vi "HXG2_PIDs.vi"(6 "PID Ctrls":T1, 7 "Analog In":T2, 8 "error in (no error)":errorcluster, 9 "AIR-LIQ Cluster":T4 {"Liq Cluster"."Liq TEMP %" min=0.0 max=100.0 step=1.0 format="%#.1f"; "Liq Cluster"."Liq FLOW %" min=0.0 max=100.0 step=1.0 format="%#.1f"; "Liq Cluster"."TLiq °F" min=40.0 max=180.0 step=1.0 format="%#.1f"; "Liq Cluster"."Mdot lbm/hr" min=0.0 max=1000.0 step=1.0 format="%#.1f"; "Air Cluster"."Air TEMP %" min=0.0 max=100.0 step=1.0 format="%#.1f"; "Air Cluster"."Air FLOW %" min=0.0 max=100.0 step=1.0 format="%#.1f"; "Air Cluster"."Tair  °F" min=-5.0 max=100.0 step=1.0 format="%#.1f"; "Air Cluster"."CFMs" min=0.0 max=200.0 step=1.0 format="%#.1f"}, 10 "PID Cluster":T7, 11 "Calculated Values":T3) -> (0 "error out":errorcluster, 3 "PID Ctrls Out":T1)   [LabVIEW 2012]
uses:
  <vilib>/addons/control/pid/NI_PID_pid.lvlib
  <vilib>/addons/control/pid/pid.llb/PID Control Input Filter (DBL).vi
  <vilib>/addons/control/pid/pid.llb/PID Advanced (DBL).vi
  Controls/UI/HXG2_NumDisplayLarge.ctl
  Modules/EnableAirGly/HXG2enable.ctl
  <vilib>/addons/control/pid/pid.llb/PID Gain Schedule (DBL).vi
  <vilib>/addons/control/pid/pid.llb/PID Structure Conversion (DBL).vi
  Controls/HXG2_PIDctrlsOUT.ctl
  Controls/HXG2_PIDon-off.ctl
  Controls/HXG2_PIDCluster.ctl
  Controls/UI/HXG2_UI_ControlSetAir.ctl
  Controls/UI/HXG2_UI_ControlSetGly.ctl
  Controls/HXG2_AirGly-Cluster.ctl
  Controls/HXG2_Calculated.ctl
  Controls/HXG2_AnalogIn.ctl
  Controls/HXG2_AirPIDresets.ctl
  Controls/HXG2_LiqPIDresets.ctl
  Controls/HXG2_PIDgains_SchedulingArray_BasicBlock.ctl
  Controls/HXG2_PIDgains_SchedulingArray.ctl
  Controls/HXG2_PIDgains_SchedulingArrayWITHLimits.ctl
panel:
  out "PID Air Heat":dbl format="%.2f"
  out "FFAir Heat":dbl
  in  "Lheat range":cluster{"setpoint high":dbl, "setpoint low":dbl}={"setpoint high"=100.0, "setpoint low"=0.0} {"setpoint high" format="%.2f"; "setpoint low" format="%.2f"}
  in  "Lcool range":cluster{"setpoint high":dbl, "setpoint low":dbl}={"setpoint high"=100.0, "setpoint low"=0.0} {"setpoint high" format="%.2f"; "setpoint low" format="%.2f"}
  out "Current State":i32
  in  "Lflow range":cluster{"setpoint high":dbl, "setpoint low":dbl}={"setpoint high"=100.0, "setpoint low"=0.0} {"setpoint high" format="%.2f"; "setpoint low" format="%.2f"}
  in  "Aheat range":cluster{"setpoint high":dbl, "setpoint low":dbl}={"setpoint high"=100.0, "setpoint low"=0.0} {"setpoint high" format="%.2f"; "setpoint low" format="%.2f"}
  in  "Acool range":cluster{"setpoint high":dbl, "setpoint low":dbl}={"setpoint high"=100.0, "setpoint low"=0.0} {"setpoint high" format="%.2f"; "setpoint low" format="%.2f"}
  in  "Aflow range":cluster{"setpoint high":dbl, "setpoint low":dbl}={"setpoint high"=100.0, "setpoint low"=0.0} {"setpoint high" format="%.2f"; "setpoint low" format="%.2f"}
  out "dt out (s)":dbl format="%.3f"
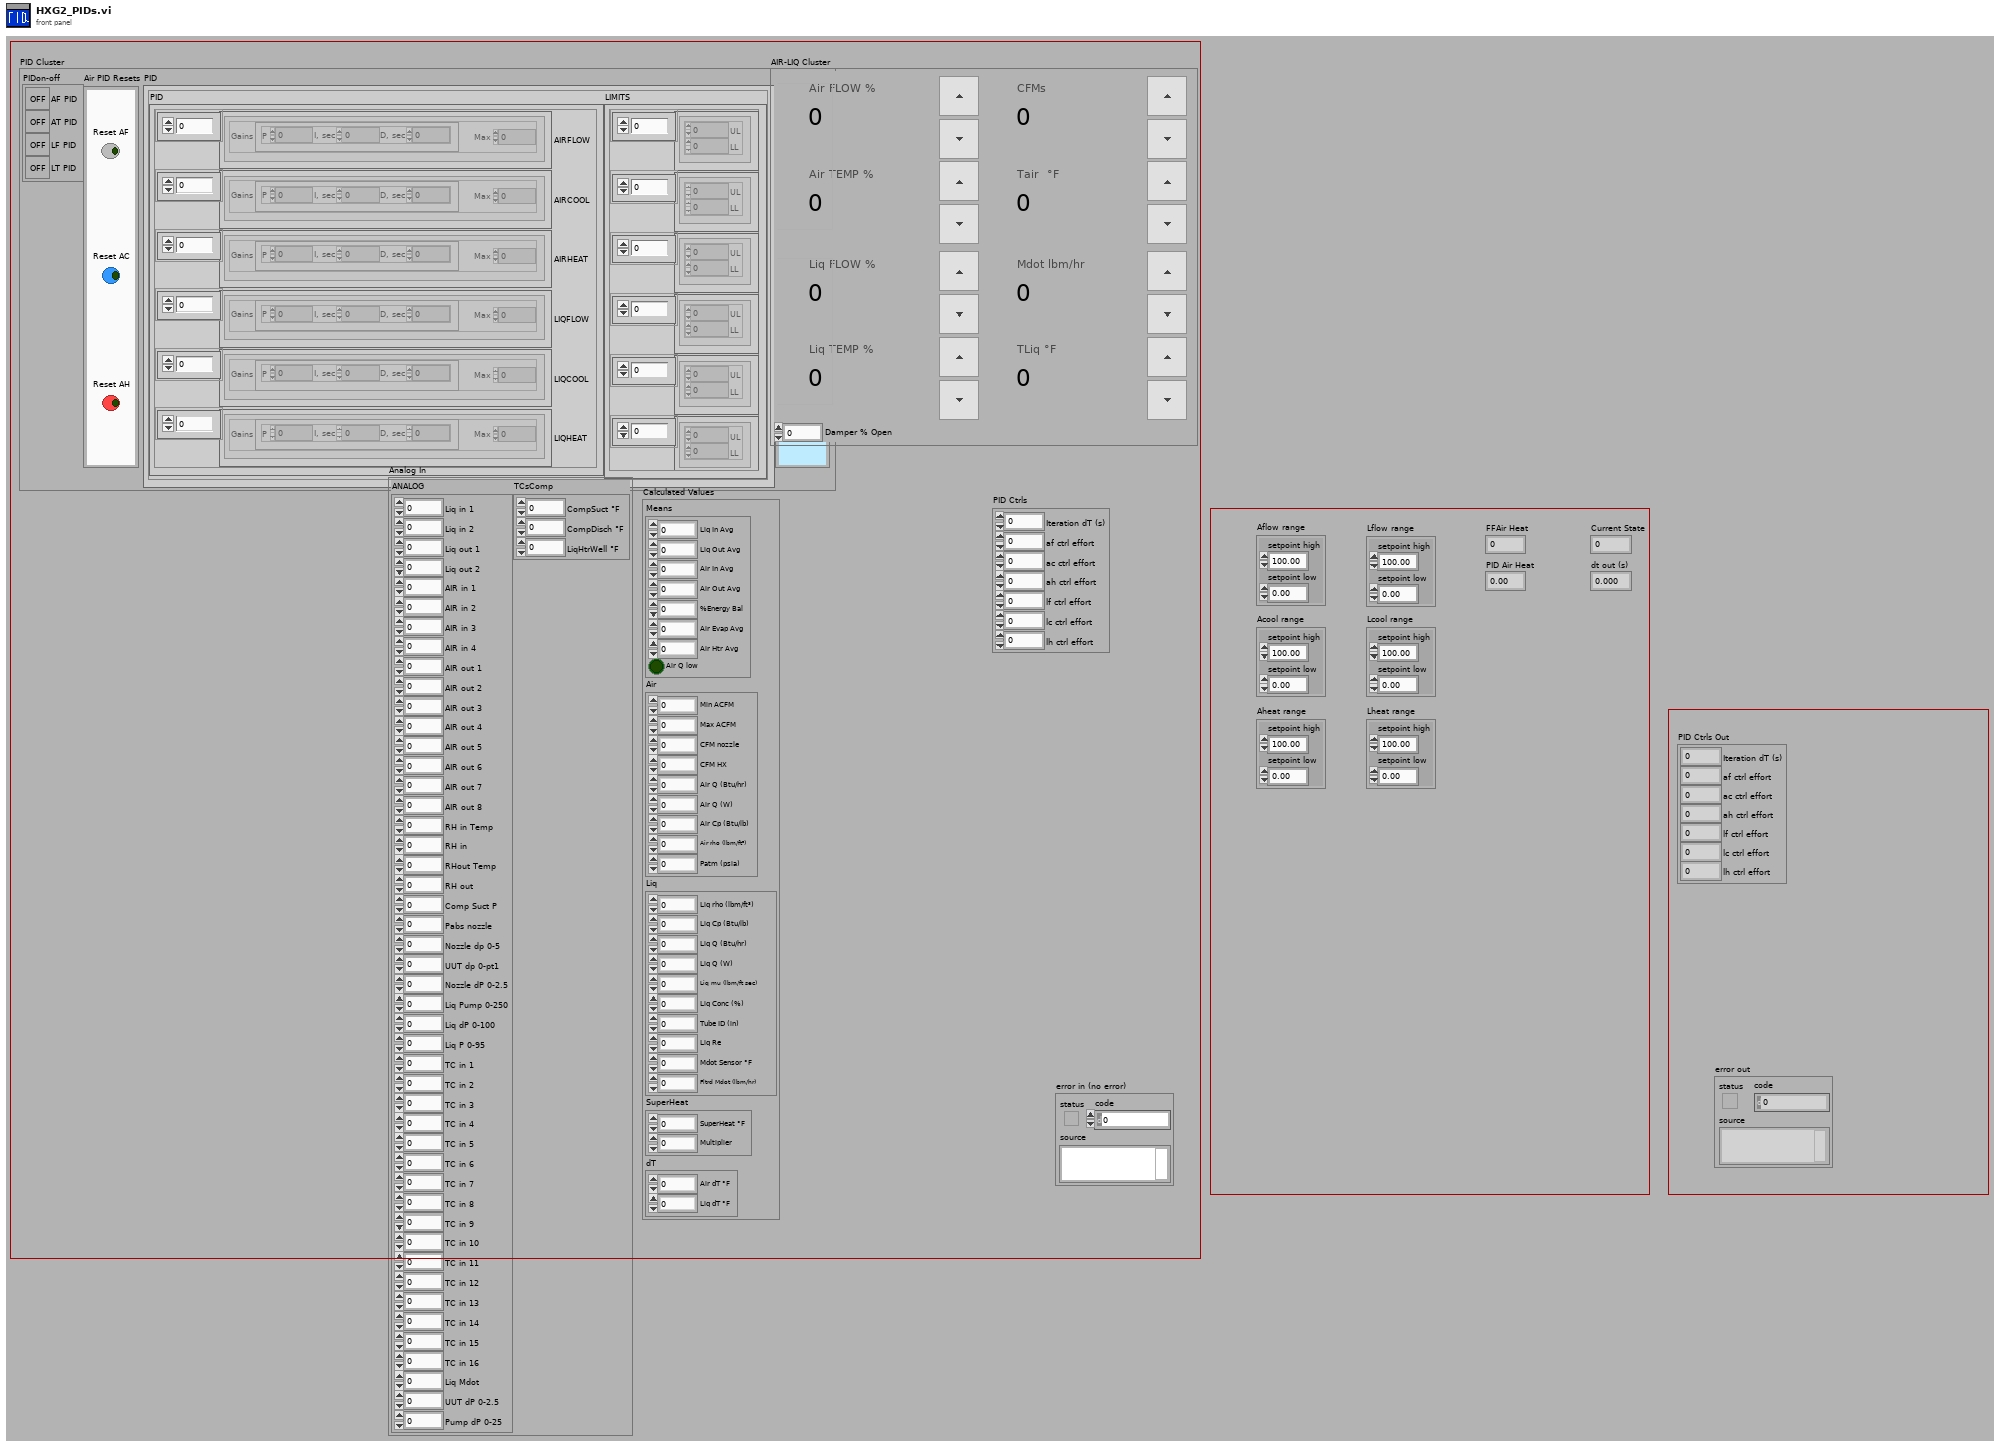
[diagram p1: front panel]
types:
  T1 = typedef "HXG2_PIDctrlsOUT.ctl" = cluster{"Iteration dT (s)":dbl, "af ctrl effort":dbl, "ac ctrl effort":dbl, "ah ctrl effort":dbl, "lf ctrl effort":dbl, "lc ctrl effort":dbl, "lh ctrl effort":dbl}
  T2 = typedef "HXG2_AnalogIn.ctl" = cluster{"ANALOG":cluster{"Liq in 1":dbl, "Liq in 2":dbl, "Liq out 1":dbl, "Liq out 2":dbl, "AIR in 1":dbl, "AIR in 2":dbl, "AIR in 3":dbl, "AIR in 4":dbl, "AIR out 1":dbl, "AIR out 2":dbl, "AIR out 3":dbl, "AIR out 4":dbl, "AIR out 5":dbl, "AIR out 6":dbl, "AIR out 7":dbl, "AIR out 8":dbl, "RH in Temp":dbl, "RH in":dbl, "RHout Temp":dbl, "RH out":dbl, "Comp Suct P":dbl, "Pabs nozzle":dbl, "Nozzle dp 0-5":dbl, "UUT dp 0-pt1":dbl, "Nozzle dP 0-2.5":dbl, "Liq Pump 0-250":dbl, "Liq dP 0-100":dbl, "Liq P 0-95":dbl, "TC in 1":dbl, "TC in 2":dbl, "TC in 3":dbl, "TC in 4":dbl, "TC in 5":dbl, "TC in 6":dbl, "TC in 7":dbl, "TC in 8":dbl, "TC in 9":dbl, "TC in 10":dbl, "TC in 11":dbl, "TC in 12":dbl, "TC in 13":dbl, "TC in 14":dbl, "TC in 15":dbl, "TC in 16":dbl, "Liq Mdot":dbl, "UUT dP 0-2.5":dbl, "Pump dP 0-25":dbl}, "TCsComp":cluster{"CompSuct °F  ":dbl, "CompDisch °F":dbl, "LiqHtrWell °F":dbl}}
  T3 = typedef "HXG2_Calculated.ctl" = cluster{"Means":cluster{"Liq In Avg":dbl, "Liq Out Avg":dbl, "Air In Avg":dbl, "Air Out Avg":dbl, "%Energy Bal":dbl, "Air Evap Avg":dbl, "Air Htr Avg":dbl, "Air Q low":bool}, "Air":cluster{"Min ACFM":dbl, "Max ACFM":dbl, "CFM nozzle":dbl, "CFM HX":dbl, "Air Q (Btu/hr)":dbl, "Air Q (W)":dbl, "Air Cp (Btu/lb)":dbl, "Air rho (lbm/ft³)":dbl, "Patm (psia)":dbl}, "Liq":cluster{"Liq rho (lbm/ft³)":dbl, "Liq Cp (Btu/lb)":dbl, "Liq Q (Btu/hr)":dbl, "Liq Q (W)":dbl, "Liq mu (lbm/ft sec)":dbl, "Liq Conc (%)":dbl, "Tube ID (in)":dbl, "Liq Re":dbl, "Mdot Sensor °F":dbl, "Fltrd Mdot (lbm/hr)":dbl}, "SuperHeat":cluster{"SuperHeat °F":dbl, "Multiplier":dbl}, "dT":cluster{"Air dT °F":dbl, "Liq dT °F":dbl}}
  T4 = typedef "HXG2_AirGly-Cluster.ctl" = cluster{"Air Cluster":T5, "Liq Cluster":T6, "Damper % Open":dbl}
  T5 = typedef "HXG2_UI_ControlSetAir.ctl" = cluster{"Air FLOW %":dbl, "Air TEMP % ":dbl, "CFMs":dbl, "Tair  °F":dbl}
  T6 = typedef "HXG2_UI_ControlSetGly.ctl" = cluster{"Liq FLOW %":dbl, "Liq TEMP % ":dbl, "Mdot lbm/hr":dbl, "TLiq °F":dbl}
  T7 = typedef "HXG2_PIDCluster.ctl" = cluster{"PIDon-off ":T8, "Air PID Resets":T9, "PID":T10, "Liq PID Resets":T13}
  T8 = typedef "HXG2_PIDon-off.ctl" = cluster{"AF PID":bool, "AT PID":bool, "LF PID":bool, "LT PID":bool}
  T9 = typedef "HXG2_AirPIDresets.ctl" = cluster{"Reset AF":bool, "Reset AC":bool, "Reset AH":bool}
  T10 = typedef "HXG2_PIDgains_SchedulingArrayWITHLimits.ctl" = cluster{"PID":T11, "LIMITS":cluster{"AIRFLOW":cluster{"UL":dbl, "LL  ":dbl}[], "AIRCOOL":cluster{"UL":dbl, "LL  ":dbl}[], "AIRHEAT":cluster{"UL":dbl, "LL  ":dbl}[], "LIQFLOW":cluster{"UL":dbl, "LL  ":dbl}[], "LIQCOOL":cluster{"UL":dbl, "LL  ":dbl}[], "LIQHEAT":cluster{"UL":dbl, "LL  ":dbl}[]}}
  T11 = typedef "HXG2_PIDgains_SchedulingArray.ctl" = cluster{"AIRFLOW":T12, "AIRCOOL":T12, "AIRHEAT":T12, "LIQFLOW":T12, "LIQCOOL":T12, "LIQHEAT":T12}
  T12 = typedef "HXG2_PIDgains_SchedulingArray_BasicBlock.ctl" = cluster{"Gains":cluster{"P":dbl, "I, sec":dbl, "D, sec":dbl}, "Max":dbl}[]
  T13 = typedef "HXG2_LiqPIDresets.ctl" = cluster{"Reset LF":bool, "Reset LC":bool, "Reset LH":bool}
  T14 = typedef "HXG2enable.ctl" = enum16{"Write Refs", "Write", "Pass"}
  T15 = typedef "HXG2_NumDisplayLarge.ctl" = dbl
  T16 = cluster{"proportional gain (Kc)":dbl, "integral time (Ti, min)":dbl, "derivative time (Td, min)":dbl}
  T17 = cluster{"Kc":dbl, "Ti, sec":dbl, "Td, sec":dbl, "UL":dbl, "LL":dbl}
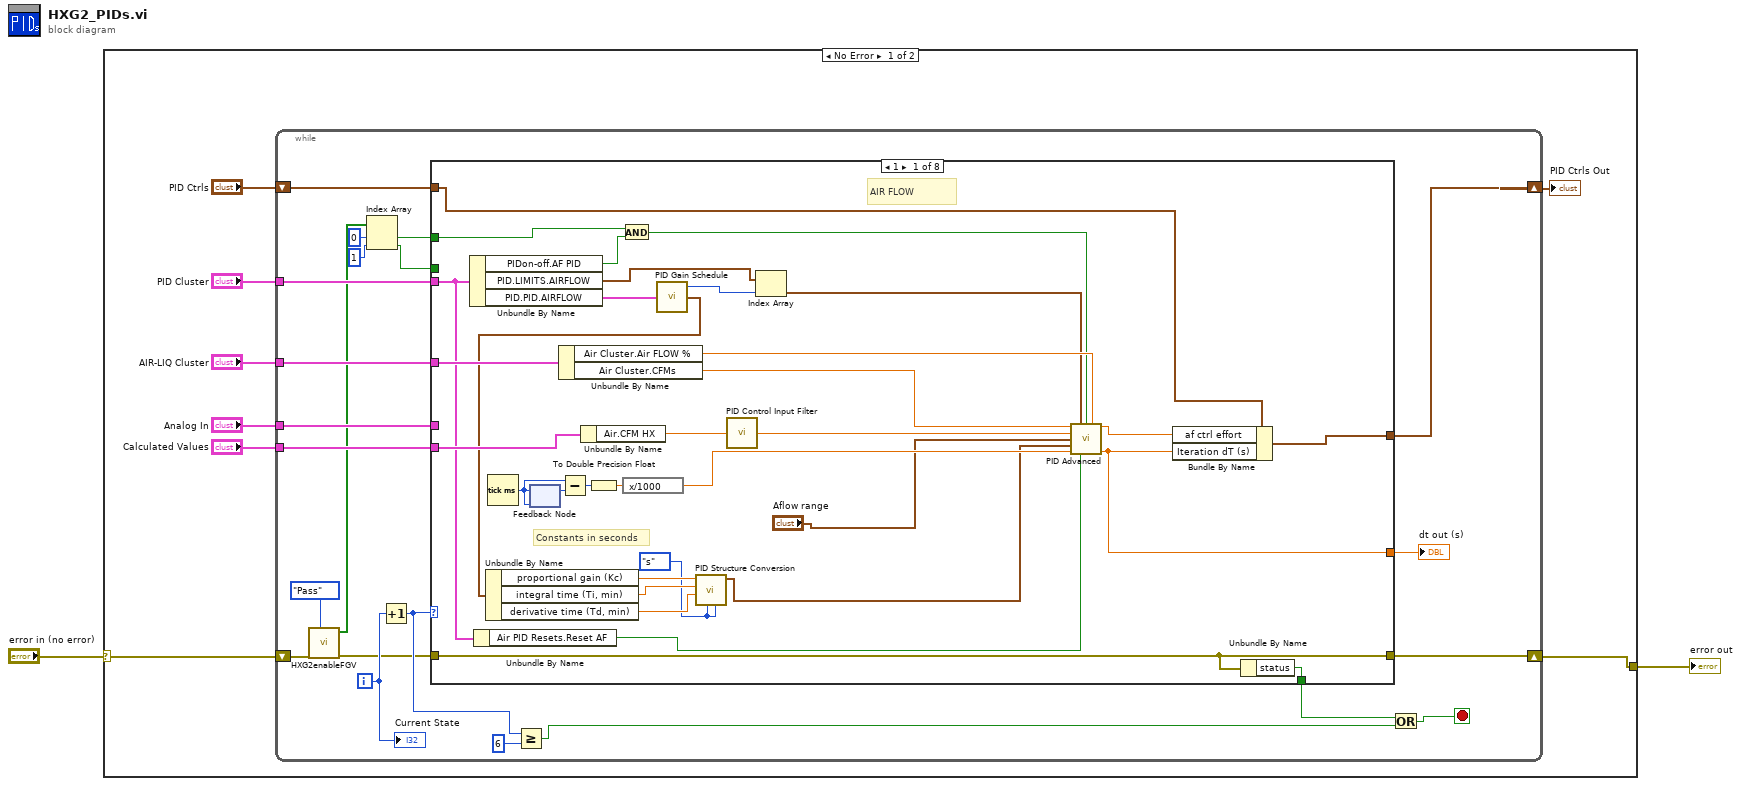
[diagram p0: block diagram]
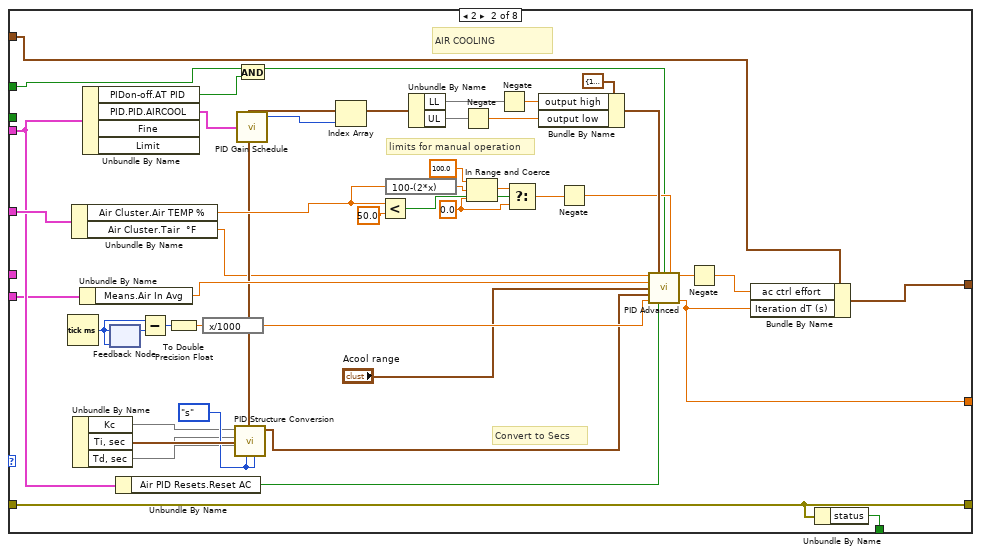
[diagram p2: hidden frame]
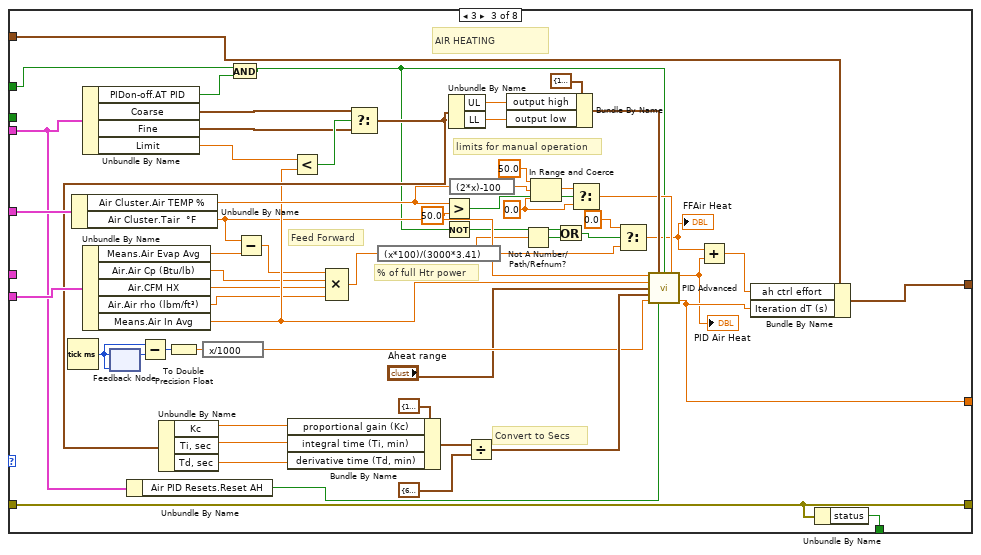
[diagram p3: hidden frame]
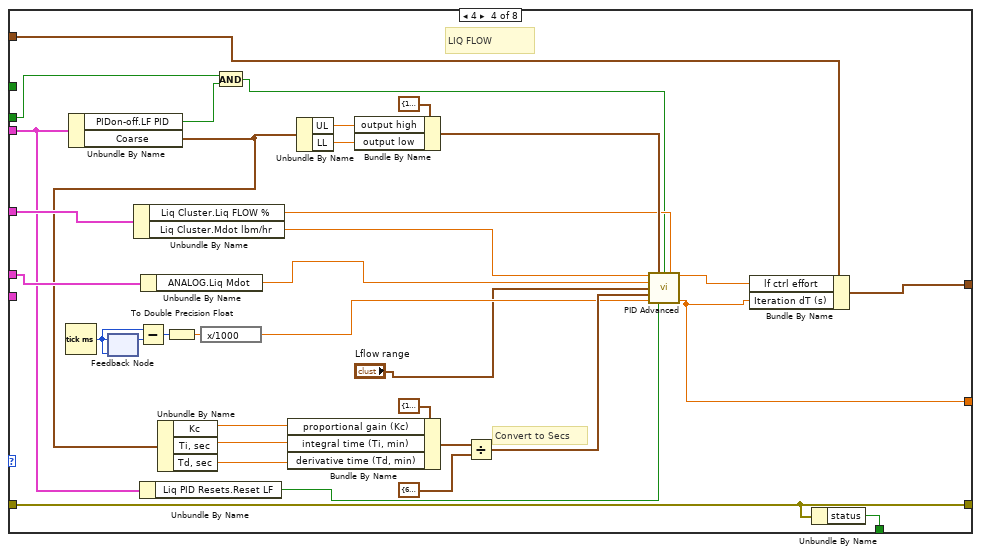
[diagram p4: hidden frame]
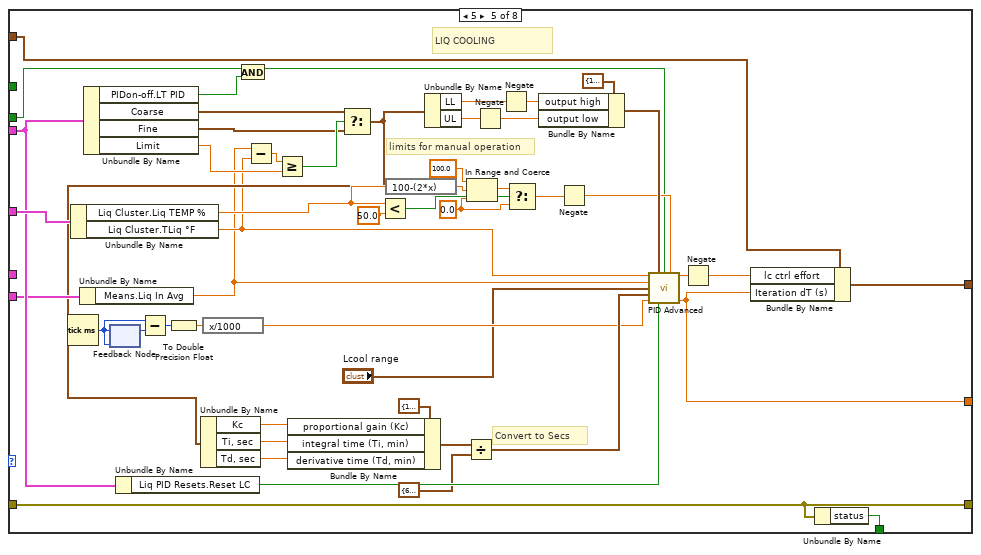
[diagram p5: hidden frame]
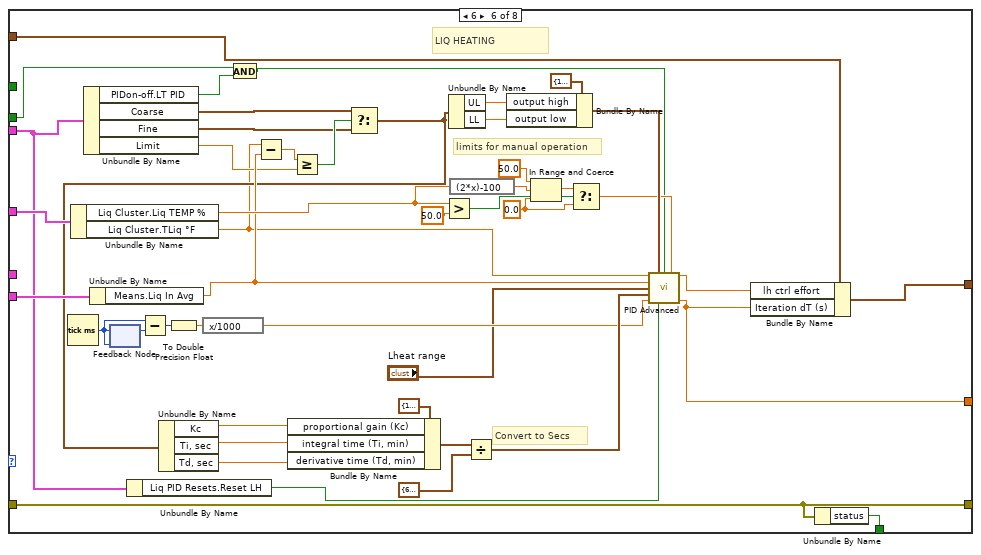
[diagram p6: hidden frame]
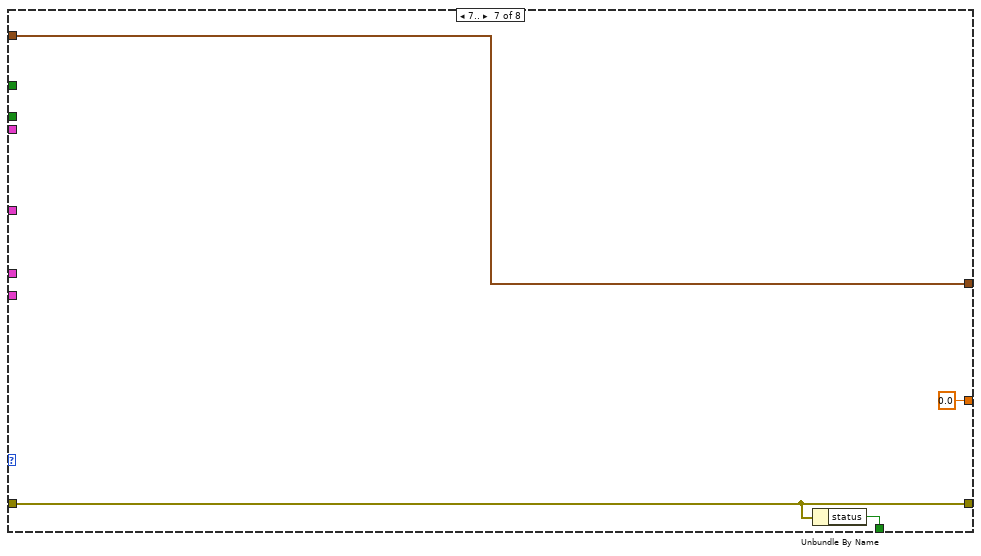
[diagram p7: hidden frame]
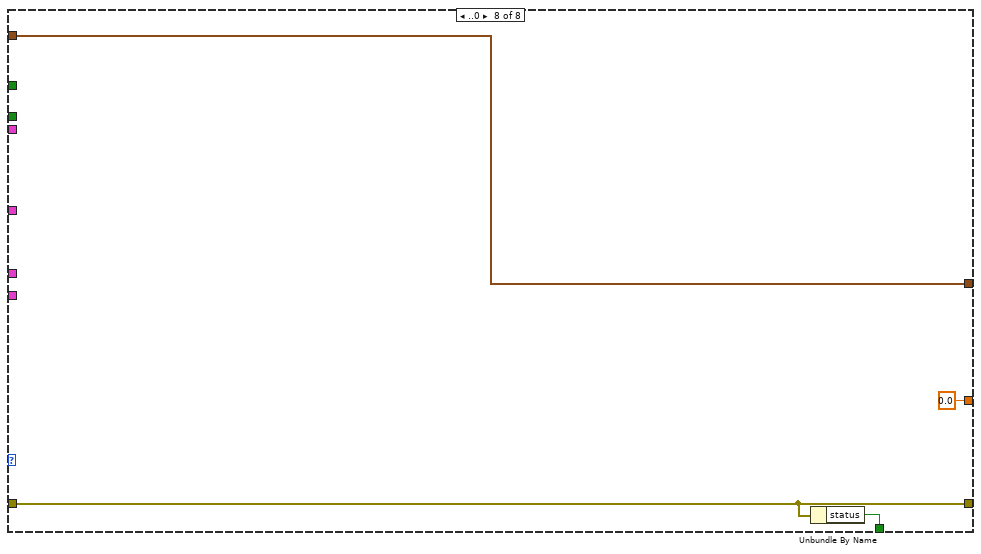
[diagram p8: hidden frame]
diagram:
  n1 = case shown="No Error" "error in (no error)" {
    selector: "error in (no error)" -> [w10 w307]
    tunnel: [w9 w307] -> w2
    frame No Error {
      n2 = while {
        tunnel: "AIR-LIQ Cluster" -> [w31]
        tunnel: "Analog In" -> [w30]
        tunnel: "PID Cluster" -> [w32]
        tunnel: "Calculated Values" -> [w29]
        shift-right: [w24] -> w3
        shift-left: "PID Ctrls" -> [w25]
        shift-right: [w11] -> w9
        shift-left: w10 -> [w19]
        i -> [w22]
        stop <- w26 stop-if-true
        n3 = call "HXG2enableFGV.vi"("ENABLE Ctrl"=HXG2enable."Pass", "error in (no error)"=w19) -> ("error out"=w18:errorcluster, "Air-Liq Out"=w16:bool[])  [unwired: 7 in, 1 out]
        n4 = Index Array(array=w16, index #1=0 ("index"), index #2=1 ("index")) -> (element #1=w13:bool, element #2=w12:bool)
        n5 = Increment(x=w22) -> (x+1=w20:i32)
        n6 = case shown="1" w20 {
          tunnel: w32 -> [w48 w107 w139 w175 w249 w267 _ _]
          tunnel: w18 -> [w51 w88 w141 w180 w226 w269 w299 w303]
          tunnel: [w51 w88 w141 w180 w226 w269 w299 w303] -> w11
          tunnel: w31 -> [w65 w108 w164 w200 w250 w294 _ _]
          tunnel: w30 -> [_ _ _ w184 _ _ _ _]
          tunnel: w25 -> [w49 w87 w140 w179 w225 w268 w301 w305]
          tunnel: w29 -> [w63 w96 w149 _ w234 w277 _ _]
          tunnel: [w59 w105 w156 w190 w243 w286 w301 w305] -> w24
          tunnel: [w46 w85 w131 w169 w209 w255 0.0 ("dt out (s)") 0.0 ("dt out (s)")] -> w23
          tunnel: [w50 w89 w142 w181 w227 w270 w300 w304] -> w21
          tunnel: w13 -> [w45 w82 w137 _ _ _ _ _]
          tunnel: w12 -> [_ _ _ w173 w210 w256 _ _]
          frame 1 {
            w34 = enum16{"min", "s"}."s" ("integral unit")
            # "Constants in seconds"
            # "AIR FLOW"
            n7 = Unbundle By Name(w48) -> ("PIDon-off.AF PID"=w44:bool, "PID.LIMITS.AIRFLOW"=w40:cluster{"UL":dbl, "LL  ":dbl}[], "PID.PID.AIRFLOW"=w42:T12)
            n8 = Unbundle By Name(w48) -> ("Air PID Resets.Reset AF"=w47:bool)
            n9 = Tick Count (ms)() -> (millisecond timer value=w56:u32)
            n10 = feedback #1(w56) -> (w58:u32)
            n11 = feedback-in #1(w56) -> ()
            n12 = Unbundle By Name(w65) -> ("Air Cluster.Air FLOW %"=w64:dbl, "Air Cluster.CFMs"=w60:dbl)
            n13 = Subtract(x=w56, y=w58) -> (x-y=w57:u32)
            n14 = Unbundle By Name(w63) -> ("Air.CFM HX"=w62:dbl)
            n15 = To Double Precision Float(number=w57) -> (double precision float=w55:dbl)
            n16 = And(x=w45, y=w44) -> (x .and. y?=w43:bool)
            n17 = expression code="x/1000"(w55) -> (w54:dbl)
            n18 = call-poly <vilib>:"PID Gain Schedule.vi"("PID gain schedule"=w42) -> ("PID gains out"=w41:T16, "index out"=w39:i32)  [unwired: 3 in]
            n19 = Unbundle By Name(w41) -> ("proportional gain (Kc)"=w37:dbl, "integral time (Ti, min)"=w36:dbl, "derivative time (Td, min)"=w35:dbl)
            n20 = call-poly <vilib>:"PID Structure Conversion.vi"("derivative unit"=w34, "integral unit"=w34, "derivative"=w35, "integral"=w36, "proportional"=w37) -> ("PID gains"=w33:T16)  [unwired: 6 in]
            n21 = call-poly <vilib>:"PID Control Input Filter.vi"("input"=w62) -> ("output"=w61:dbl)  [unwired: 4 in]
            n22 = Index Array(array=w40, index=w39) -> (element=w38:cluster{"UL":dbl, "LL  ":dbl})
            n23 = call-poly <vilib>:"PID Advanced.vi"("setpoint"=w60, "output range"=w38, "auto? (T)"=w43, "manual control"=w64, "process variable"=w61, "setpoint range"="Aflow range", "PID gains"=w33, "dt (s)"=w54, "reinitialize? (F)"=w47) -> ("output"=w53:dbl, "dt out (s)"=w46:dbl)  [unwired: 5 in]
            n24 = Bundle By Name(cluster=w49, "af ctrl effort"=w53, "Iteration dT (s)"=w46) -> (w59:T1)
            n25 = Unbundle By Name(w51) -> ("status"=w50:bool)
          }
          frame 2 {
            w72 = enum16{"min", "s"}."s" ("integral unit")
            w103 = T15 0.0 ("lower limit")
            # "limits for manual operation"
            # "Convert to Secs"
            # "AIR COOLING"
            n26 = Tick Count (ms)() -> (millisecond timer value=w93:u32)
            n27 = Unbundle By Name(w108) -> ("Air Cluster.Air TEMP %"=w98:dbl, "Air Cluster.Tair  °F"=w73:dbl)
            n28 = Unbundle By Name() -> (w78:T17, "Kc"=w71, "Ti, sec"=w70, "Td, sec"=w69)
            n29 = Unbundle By Name(w96) -> ("Means.Air In Avg"=w79:dbl)
            n30 = Unbundle By Name(w107) -> ("PIDon-off.AT PID"=w81:bool, "PID.PID.AIRCOOL"=w66:T12)  [unwired: 2 out]
            n31 = feedback #2(w93) -> (w95:u32)
            n32 = feedback-in #2(w93) -> ()
            n33 = Unbundle By Name(w107) -> ("Air PID Resets.Reset AC"=w106:bool)
            n34 = Subtract(x=w93, y=w95) -> (x-y=w94:u32)
            n35 = To Double Precision Float(number=w94) -> (double precision float=w92:dbl)
            n36 = expression code="x/1000"(w92) -> (w91:dbl)
            n37 = call-poly <vilib>:"PID Structure Conversion.vi"("derivative unit"=w72, "integral unit"=w72, "derivative"=w69, "integral"=w70, "proportional"=w71) -> ("PID gains"=w68:T16)  [unwired: 6 in]
            n38 = call-poly <vilib>:"PID Gain Schedule.vi"("PID gain schedule"=w66) -> ("index out"=w67:i32)  [unwired: 3 in, 1 out]
            n39 = And(x=w82, y=w81) -> (x .and. y?=w80:bool)
            n40 = Index Array(index=w67) -> ()  [unwired: 1 in, 1 out]
            n41 = Less?(x=w98, y=T15 50.0) -> (x < y?=w104:bool)
            n42 = expression code="100-(2*x)"(w98) -> (w101:dbl)
            n43 = Unbundle By Name(w78) -> ("LL"=w84, "UL"=w83)
            n44 = Negate(x=w83) -> (-x=w75:dbl)
            n45 = In Range and Coerce(upper limit=T15 100.0, x=w101, lower limit=w103) -> (coerced(x)=w100:T15)  [unwired: 1 out]
            n46 = Negate(x=w84) -> (-x=w74:dbl)
            n47 = Select(t=w100, s=w104, f=w103) -> (s? t:f=w97:T15)
            n48 = Bundle By Name(cluster=cluster{"output high":dbl, "output low":dbl} {"output high"=100.0, "output low"=-100.0} ("output range"), "output high"=w74, "output low"=w75) -> (w109:cluster{"output high":dbl, "output low":dbl})
            n49 = Negate(x=w97) -> (-x=w86:T15)
            n50 = call-poly <vilib>:"PID Advanced.vi"("setpoint"=w73, "output range"=w109, "auto? (T)"=w80, "manual control"=w86, "process variable"=w79, "setpoint range"="Acool range", "PID gains"=w68, "dt (s)"=w91, "reinitialize? (F)"=w106) -> ("output"=w77:dbl, "dt out (s)"=w85:dbl)  [unwired: 5 in]
            n51 = Negate(x=w77) -> (-x=w76:dbl)
            n52 = Bundle By Name(cluster=w87, "ac ctrl effort"=w76, "Iteration dT (s)"=w85) -> (w105:T1)
            n53 = Unbundle By Name(w88) -> ("status"=w89:bool)
          }
          frame 3 {
            w119 = T15 0.0 ("lower limit")
            # "% of full Htr power"
            # "Feed Forward"
            # "limits for manual operation"
            # "Convert to Secs"
            # "AIR HEATING"
            n54 = Tick Count (ms)() -> (millisecond timer value=w146:u32)
            n55 = Unbundle By Name(w164) -> ("Air Cluster.Air TEMP %"=w150:dbl, "Air Cluster.Tair  °F"=w124:dbl)
            n56 = Unbundle By Name(w139) -> ("PIDon-off.AT PID"=w136:bool, "Coarse"=w134:T17, "Fine"=w133:T17, "Limit"=w130:dbl)
            n57 = Unbundle By Name(w149) -> ("Means.Air Evap Avg"=w125:dbl, "Air.Air Cp (Btu/lb)"=w128:dbl, "Air.CFM HX"=w127:dbl, "Air.Air rho (lbm/ft³)"=w126:dbl, "Means.Air In Avg"=w129:dbl)
            n58 = feedback #3(w146) -> (w148:u32)
            n59 = feedback-in #3(w146) -> ()
            n60 = Unbundle By Name(w139) -> ("Air PID Resets.Reset AH"=w138:bool)
            n61 = Subtract(x=w146, y=w148) -> (x-y=w147:u32)
            n62 = To Double Precision Float(number=w147) -> (double precision float=w145:dbl)
            n63 = expression code="x/1000"(w145) -> (w144:dbl)
            n64 = And(x=w137, y=w136) -> (x .and. y?=w117:bool)
            n65 = Subtract(x=w124, y=w125) -> (x-y=w123:dbl)
            n66 = Less?(x=w130, y=w129) -> (x < y?=w135:bool)
            n67 = Compound Arithmetic op=MULTIPLY(w123, w128, w127, w126) -> (w113:dbl)
            n68 = Select(t=w134, s=w135, f=w133) -> (s? t:f=w132:T17)
            n69 = Unbundle By Name(w132) -> ("Kc"=w162:dbl, "Ti, sec"=w161:dbl, "Td, sec"=w160:dbl)
            n70 = Bundle By Name(cluster=T16 {"proportional gain (Kc)"=1.0, "integral time (Ti, min)"=0.01, "derivative time (Td, min)"=0.0} ("PID gains"), "proportional gain (Kc)"=w162, "integral time (Ti, min)"=w161, "derivative time (Td, min)"=w160) -> (w159:T16)
            n71 = expression code="(x*100)/(3000*3.41)"(w113) -> (w112:dbl)
            n72 = Greater?(x=w150, y=T15 50.0) -> (0:w155:bool)
            n73 = Not(x=w117) -> (.not. x?=w114:bool)
            n74 = Unbundle By Name(w132) -> ("UL"=w167:dbl, "LL"=w168:dbl)
            n75 = expression code="(2*x)-100"(w150) -> (w153:dbl)
            n76 = Divide(x=w159, y=T16 {"proportional gain (Kc)"=60.0, "integral time (Ti, min)"=60.0, "derivative time (Td, min)"=60.0}) -> (x/y=w157:T16)
            n77 = Bundle By Name(cluster=cluster{"output high":dbl, "output low":dbl} {"output high"=100.0, "output low"=-100.0} ("output range"), "output high"=w167, "output low"=w168) -> (w165:cluster{"output high":dbl, "output low":dbl})
            n78 = Not A Number/Path/Refnum?(number/path/refnum=w112) -> (NaN/Path/Refnum?=w116:bool)
            n79 = In Range and Coerce(upper limit=T15 50.0, x=w153, lower limit=w119) -> (coerced(x)=w152:T15)  [unwired: 1 out]
            n80 = Or(x=w114, y=w116) -> (x .or. y?=w115:bool)
            n81 = Select(t=w152, s=w155, f=w119) -> (s? t:f=w120:T15)
            n82 = Select(t=0.0, s=w115, f=w112) -> (s? t:f=w111:dbl)
            "FFAir Heat" <- w111
            n83 = call-poly <vilib>:"PID Advanced.vi"("setpoint"=w124, "output range"=w165, "auto? (T)"=w117, "manual control"=w120, "process variable"=w129, "setpoint range"="Aheat range", "PID gains"=w157, "dt (s)"=w144, "reinitialize? (F)"=w138) -> ("output"=w122:dbl, "dt out (s)"=w131:dbl)  [unwired: 5 in]
            "PID Air Heat" <- w122
            n84 = Add(x=w111, y=w122) -> (x+y=w121:dbl)
            n85 = Bundle By Name(cluster=w140, "ah ctrl effort"=w121, "Iteration dT (s)"=w131) -> (w156:T1)
            n86 = Unbundle By Name(w141) -> ("status"=w142:bool)
          }
          frame 4 {
            # "Convert to Secs"
            # "LIQ FLOW"
            n87 = Tick Count (ms)() -> (millisecond timer value=w187:u32)
            n88 = Unbundle By Name(w175) -> ("PIDon-off.LF PID"=w172:bool, "Coarse"=w170:T17)
            n89 = feedback #4(w187) -> (w189:u32)
            n90 = feedback-in #4(w187) -> ()
            n91 = Unbundle By Name(w200) -> ("Liq Cluster.Liq FLOW %"=w199:dbl, "Liq Cluster.Mdot lbm/hr"=w191:dbl)
            n92 = Subtract(x=w187, y=w189) -> (x-y=w188:u32)
            n93 = Unbundle By Name(w175) -> ("Liq PID Resets.Reset LF"=w174:bool)
            n94 = Unbundle By Name(w184) -> ("ANALOG.Liq Mdot"=w178:dbl)
            n95 = Unbundle By Name(w170) -> ("Kc"=w197:dbl, "Ti, sec"=w196:dbl, "Td, sec"=w195:dbl)
            n96 = To Double Precision Float(number=w188) -> (double precision float=w186:dbl)
            n97 = expression code="x/1000"(w186) -> (w185:dbl)
            n98 = And(x=w173, y=w172) -> (x .and. y?=w171:bool)
            n99 = Bundle By Name(cluster=T16 {"proportional gain (Kc)"=1.0, "integral time (Ti, min)"=0.01, "derivative time (Td, min)"=0.0} ("PID gains"), "proportional gain (Kc)"=w197, "integral time (Ti, min)"=w196, "derivative time (Td, min)"=w195) -> (w194:T16)
            n100 = Unbundle By Name(w170) -> ("UL"=w177:dbl, "LL"=w176:dbl)
            n101 = Bundle By Name(cluster=cluster{"output high":dbl, "output low":dbl} {"output high"=100.0, "output low"=-100.0} ("output range"), "output high"=w177, "output low"=w176) -> (w201:cluster{"output high":dbl, "output low":dbl})
            n102 = Divide(x=w194, y=T16 {"proportional gain (Kc)"=60.0, "integral time (Ti, min)"=60.0, "derivative time (Td, min)"=60.0}) -> (x/y=w192:T16)
            n103 = call-poly <vilib>:"PID Advanced.vi"("setpoint"=w191, "output range"=w201, "auto? (T)"=w171, "manual control"=w199, "process variable"=w178, "setpoint range"="Lflow range", "PID gains"=w192, "dt (s)"=w185, "reinitialize? (F)"=w174) -> ("output"=w183:dbl, "dt out (s)"=w169:dbl)  [unwired: 5 in]
            n104 = Bundle By Name(cluster=w179, "lf ctrl effort"=w183, "Iteration dT (s)"=w169) -> (w190:T1)
            n105 = Unbundle By Name(w180) -> ("status"=w181:bool)
          }
          frame 5 {
            w241 = T15 0.0 ("lower limit")
            # "limits for manual operation"
            # "Convert to Secs"
            # "LIQ COOLING"
            n106 = Tick Count (ms)() -> (millisecond timer value=w231:u32)
            n107 = Unbundle By Name(w250) -> ("Liq Cluster.Liq TEMP %"=w236:dbl, "Liq Cluster.TLiq °F"=w206:dbl)
            n108 = Unbundle By Name(w234) -> ("Means.Liq In Avg"=w204:dbl)
            n109 = Unbundle By Name(w249) -> ("PIDon-off.LT PID"=w218:bool, "Coarse"=w213:T17, "Fine"=w212:T17, "Limit"=w214:dbl)
            n110 = feedback #5(w231) -> (w233:u32)
            n111 = feedback-in #5(w231) -> ()
            n112 = Unbundle By Name(w249) -> ("Liq PID Resets.Reset LC"=w248:bool)
            n113 = Subtract(x=w231, y=w233) -> (x-y=w232:u32)
            n114 = To Double Precision Float(number=w232) -> (double precision float=w230:dbl)
            n115 = expression code="x/1000"(w230) -> (w229:dbl)
            n116 = And(x=w210, y=w218) -> (x .and. y?=w217:bool)
            n117 = Subtract(x=w204, y=w206) -> (x-y=w216:dbl)
            n118 = Greater Or Equal?(x=w216, y=w214) -> (x >= y?=w215:bool)
            n119 = Select(t=w213, s=w215, f=w212) -> (s? t:f=w211:T17)
            n120 = Unbundle By Name(w211) -> ("Kc"=w223:dbl, "Ti, sec"=w222:dbl, "Td, sec"=w221:dbl)
            n121 = Bundle By Name(cluster=T16 {"proportional gain (Kc)"=1.0, "integral time (Ti, min)"=0.01, "derivative time (Td, min)"=0.0} ("PID gains"), "proportional gain (Kc)"=w223, "integral time (Ti, min)"=w222, "derivative time (Td, min)"=w221) -> (w246:T16)
            n122 = Less?(x=w236, y=T15 50.0) -> (x < y?=w242:bool)
            n123 = expression code="100-(2*x)"(w236) -> (w239:dbl)
            n124 = Unbundle By Name(w211) -> ("LL"=w220:dbl, "UL"=w219:dbl)
            n125 = Divide(x=w246, y=T16 {"proportional gain (Kc)"=60.0, "integral time (Ti, min)"=60.0, "derivative time (Td, min)"=60.0}) -> (x/y=w244:T16)
            n126 = In Range and Coerce(upper limit=T15 100.0, x=w239, lower limit=w241) -> (coerced(x)=w238:T15)  [unwired: 1 out]
            n127 = Negate(x=w219) -> (-x=w207:dbl)
            n128 = Negate(x=w220) -> (-x=w208:dbl)
            n129 = Select(t=w238, s=w242, f=w241) -> (s? t:f=w235:T15)
            n130 = Bundle By Name(cluster=cluster{"output high":dbl, "output low":dbl} {"output high"=100.0, "output low"=-100.0} ("output range"), "output high"=w208, "output low"=w207) -> (w251:cluster{"output high":dbl, "output low":dbl})
            n131 = Negate(x=w235) -> (-x=w224:T15)
            n132 = call-poly <vilib>:"PID Advanced.vi"("setpoint"=w206, "output range"=w251, "auto? (T)"=w217, "manual control"=w224, "process variable"=w204, "setpoint range"="Lcool range", "PID gains"=w244, "dt (s)"=w229, "reinitialize? (F)"=w248) -> ("output"=w205:dbl, "dt out (s)"=w209:dbl)  [unwired: 5 in]
            n133 = Negate(x=w205) -> (-x=w203:dbl)
            n134 = Bundle By Name(cluster=w225, "lc ctrl effort"=w203, "Iteration dT (s)"=w209) -> (w243:T1)
            n135 = Unbundle By Name(w226) -> ("status"=w227:bool)
          }
          frame 6 {
            w284 = T15 0.0 ("lower limit")
            # "limits for manual operation"
            # "Convert to Secs"
            # "LIQ HEATING"
            n136 = Tick Count (ms)() -> (millisecond timer value=w274:u32)
            n137 = Unbundle By Name(w294) -> ("Liq Cluster.Liq TEMP %"=w279:dbl, "Liq Cluster.TLiq °F"=w254:dbl)
            n138 = Unbundle By Name(w267) -> ("PIDon-off.LT PID"=w265:bool, "Coarse"=w260:T17, "Fine"=w259:T17, "Limit"=w257:dbl)
            n139 = Unbundle By Name(w277) -> ("Means.Liq In Avg"=w261:dbl)
            n140 = feedback #6(w274) -> (w276:u32)
            n141 = feedback-in #6(w274) -> ()
            n142 = Unbundle By Name(w267) -> ("Liq PID Resets.Reset LH"=w266:bool)
            n143 = Subtract(x=w274, y=w276) -> (x-y=w275:u32)
            n144 = To Double Precision Float(number=w275) -> (double precision float=w273:dbl)
            n145 = expression code="x/1000"(w273) -> (w272:dbl)
            n146 = And(x=w256, y=w265) -> (x .and. y?=w264:bool)
            n147 = Subtract(x=w254, y=w261) -> (x-y=w263:dbl)
            n148 = Greater Or Equal?(x=w263, y=w257) -> (x >= y?=w262:bool)
            n149 = Select(t=w260, s=w262, f=w259) -> (s? t:f=w258:T17)
            n150 = Unbundle By Name(w258) -> ("Kc"=w292:dbl, "Ti, sec"=w291:dbl, "Td, sec"=w290:dbl)
            n151 = Bundle By Name(cluster=T16 {"proportional gain (Kc)"=1.0, "integral time (Ti, min)"=0.01, "derivative time (Td, min)"=0.0} ("PID gains"), "proportional gain (Kc)"=w292, "integral time (Ti, min)"=w291, "derivative time (Td, min)"=w290) -> (w289:T16)
            n152 = Greater?(x=w279, y=T15 50.0) -> (0:w285:bool)
            n153 = Unbundle By Name(w258) -> ("UL"=w297:dbl, "LL"=w298:dbl)
            n154 = expression code="(2*x)-100"(w279) -> (w282:dbl)
            n155 = Divide(x=w289, y=T16 {"proportional gain (Kc)"=60.0, "integral time (Ti, min)"=60.0, "derivative time (Td, min)"=60.0}) -> (x/y=w287:T16)
            n156 = Bundle By Name(cluster=cluster{"output high":dbl, "output low":dbl} {"output high"=100.0, "output low"=-100.0} ("output range"), "output high"=w297, "output low"=w298) -> (w295:cluster{"output high":dbl, "output low":dbl})
            n157 = In Range and Coerce(upper limit=T15 50.0, x=w282, lower limit=w284) -> (coerced(x)=w281:T15)  [unwired: 1 out]
            n158 = Select(t=w281, s=w285, f=w284) -> (s? t:f=w278:T15)
            n159 = call-poly <vilib>:"PID Advanced.vi"("setpoint"=w254, "output range"=w295, "auto? (T)"=w264, "manual control"=w278, "process variable"=w261, "setpoint range"="Lheat range", "PID gains"=w287, "dt (s)"=w272, "reinitialize? (F)"=w266) -> ("output"=w253:dbl, "dt out (s)"=w255:dbl)  [unwired: 5 in]
            n160 = Bundle By Name(cluster=w268, "lh ctrl effort"=w253, "Iteration dT (s)"=w255) -> (w286:T1)
            n161 = Unbundle By Name(w269) -> ("status"=w270:bool)
          }
          frame 7.. {
            n162 = Unbundle By Name(w299) -> ("status"=w300:bool)
          }
          frame ..0 {
            n163 = Unbundle By Name(w303) -> ("status"=w304:bool)
          }
        }
        "dt out (s)" <- w23
        n164 = Greater Or Equal?(x=w20, y=6) -> (x >= y?=w27:bool)
        n165 = Or(x=w21, y=w27) -> (x .or. y?=w26:bool)
        "Current State" <- w22
      }
      "PID Ctrls Out" <- w3
    }
    frame Error {
    }
  }
  "error out" <- w2
